vi "New File.vi"(8 "error in":errorcluster, 11 "File Observer in":refnum<class "File Observer.lvclass">) -> (0 "error out":errorcluster, 2 "Exceeded":bool, 3 "File Observer out":refnum<class "File Observer.lvclass">)   [LabVIEW 2015, in "File Observer.lvclass"]
doc: "Housekeeping to see if the current file has exceeded the maximum file size indicated by the caller. If it has, the variable Exceeded == TRUE."
uses:
  File Observer.lvclass
  File Observer.lvclass/File Observer.ctl
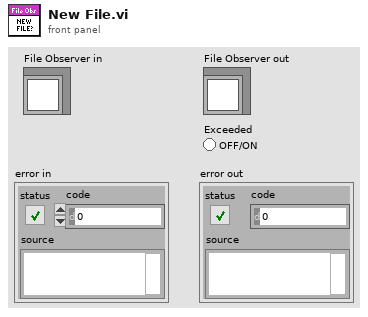
[diagram p1: front panel]
types:
  T1 = typedef "LVDateTimeRec.ctl" = cluster{"fractional second":dbl, "second":i32, "minute":i32, "hour":i32, "day of month":i32, "month":i32, "year":i32, "day of week":i32, "day of year":i32, "DST":i32}
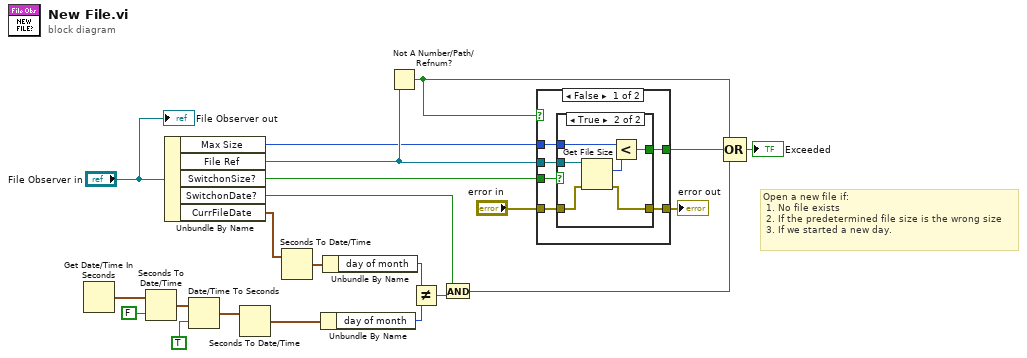
[diagram p0: block diagram]
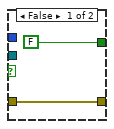
[diagram p2: hidden frame]
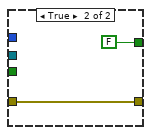
[diagram p3: hidden frame]
diagram:
  # "Open a new file if:\n 1. No file exists\n 2. If the predetermined file size is the wrong size\n 3. If we started a new day."
  n1 = Get Date/Time In Seconds() -> (seconds since 1Jan1904=w7:timestamp)
  n2 = Seconds To Date/Time(time stamp (now)=w7, to UTC (F)=FALSE) -> (date time rec=w4:T1)
  n3 = Unbundle By Name("File Observer in") -> ("Max Size"=w19:i64, "File Ref"=w20:refnum<file>, "SwitchonSize?"=w17:bool, "SwitchonDate?"=w14:bool, "CurrFileDate"=w13:timestamp)
  n4 = Date/Time To Seconds(1:TRUE ("is UTC (F)"), 2:w4) -> (0:w3:timestamp)
  n5 = Seconds To Date/Time(time stamp (now)=w3) -> (date time rec=w2:T1)  [unwired: 1 in]
  n6 = Seconds To Date/Time(time stamp (now)=w13) -> (date time rec=w12:T1)  [unwired: 1 in]
  n7 = Unbundle By Name(w2) -> ("day of month"=w11:i32)
  n8 = Unbundle By Name(w12) -> ("day of month"=w10:i32)
  n9 = Not A Number/Path/Refnum?(number/path/refnum=w20) -> (NaN/Path/Refnum?=w1:bool)
  n10 = Not Equal?(x=w10, y=w11) -> (x != y?=w9:bool)
  n11 = And(x=w14, y=w9) -> (x .and. y?=w8:bool)
  n12 = case shown="False" w1 {
    tunnel: [w28 w37] -> w22
    tunnel: "error in" -> [w27 w37]
    tunnel: w20 -> [w26 _]
    tunnel: w19 -> [w25 _]
    tunnel: w17 -> [w24 _]
    tunnel: [w23 FALSE] -> w16
    frame False {
      n13 = case shown="True" w24 {
        tunnel: [w30 w36] -> w28
        tunnel: w27 -> [w30 w35]
        tunnel: w26 -> [_ w34]
        tunnel: w25 -> [_ w33]
        tunnel: [FALSE w31] -> w23
        frame False {
        }
        frame True {
          n14 = Get File Size(file=w34, error in=w35) -> (size (in bytes)=w32:i64, 0:w36:errorcluster)  [unwired: 1 out]
          n15 = Less?(x=w33, y=w32) -> (x < y?=w31:bool)
        }
      }
    }
    frame True {
    }
  }
  "error out" <- w22
  n16 = Compound Arithmetic op=OR(w1, w16, w8) -> (→"Exceeded":bool)
  "File Observer out" <- "File Observer in"
